vi "Get Common Property Values.vi"(8 "Error In":errorcluster, 11 "Data Channel  Ref in":T2 format="%.0x") -> (0 "error out":errorcluster, 2 "Array Out":T1[](array[typedef]), 3 "Data Channel Ref Out":u64)   [LabVIEW 2019, in "Instrument Addon Scripting API Channels Unit Tests.lvclass"]
uses:
  Instrument Addon Scripting API Channels Unit Tests.lvclass
  <vilib>/NI VeriStand/Custom Device API/Custom Device Item Ref.ctl
  APIs/Scripting API/TypeDefs/Array Element.ctl
  Addon/Addon Shared/SubVIs/Constants.vi
  <vilib>/NI/NI VeriStand Advanced SysDef API/_SubVIs/SysDef.Search.GUIDs.vi
  APIs/Scripting API/Instrument Addon Scripting API.lvlib
  <vilib>/NI VeriStand/Custom Device API/Custom Device API.lvlib
  <vilib>/NI/NI VeriStand Advanced SysDef API/SysDef API/Advanced System Definition.lvlib
  Addon/Addon Shared/Instrument Addon Shared.lvlib
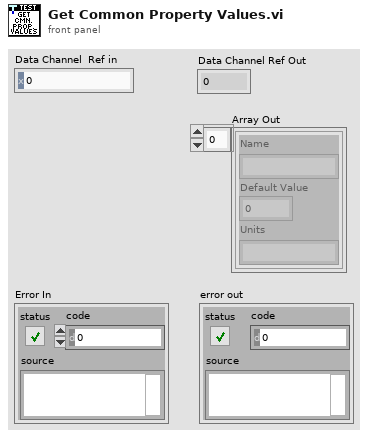
[diagram p1: front panel]
types:
  T1 = typedef "Instrument Addon Scripting API.lvlib/Array Element.ctl" = cluster{"Name":string, "Default Value":dbl, "Units":string}
  T2 = typedef "Custom Device API.lvlib/Custom Device Item Ref.ctl" = u64
  T3 = typedef "Custom Device API.lvlib/Custom Device Channel.ctl" = cluster{"Type":T4, "Units":string, "Default Value":dbl, "Faultable":bool, "Scalable":bool}
  T4 = typedef "Custom Device API.lvlib/Custom Device Channel Type.ctl" = enum16{"Input", "Output"}
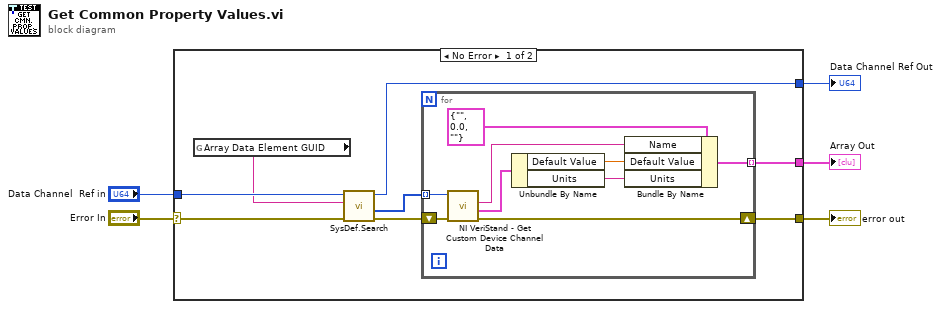
[diagram p0: block diagram]
diagram:
  n1 = case shown="No Error" "Error In" {
    selector: "Error In" -> [w7 w24]
    tunnel: "Data Channel  Ref in" -> [w13 w23]
    tunnel: [w12 _] -> w4
    tunnel: [w11 w23] -> w3
    tunnel: [w10 w24] -> w2
    frame No Error {
      n2 = global read "Constants.vi" "Array Data Element GUID"() -> (w6:string)
      n3 = call-poly <vilib>:"SysDef.Search.vi"("error in (no error)"=w7, "GUID"=w6, "nodeID"=w13) -> ("error out"=w8:errorcluster, "Values Out"=w9:u64[], "nodeID out"=w11:u64)  [unwired: 5 in, 1 out]
      n4 = for {
        shift-right: [w14] -> w10
        shift-left: w8 -> [w21]
        tunnel: w9 -> [w22] mode=indexing
        tunnel: [w15] -> w12 mode=indexing
        n5 = call <vilib>:"NI VeriStand - Get Custom Device Channel Data.vi"("error in (no error)"=w21, "Channel Ref in"=w22) -> ("error out"=w14:errorcluster, "Channel"=w18:T3, "Channel Name"=w19:string)  [unwired: 4 in, 3 out]
        n6 = Unbundle By Name(w18) -> ("Default Value"=w16:dbl, "Units"=w17:string)
        n7 = Bundle By Name(cluster=T1 {"Name"="", "Default Value"=0.0, "Units"=""} ("Array Element"), "Name"=w19, "Default Value"=w16, "Units"=w17) -> (w15:T1)
      }
    }
    frame Error {
    }
  }
  "Array Out" <- w4
  "Data Channel Ref Out" <- w3
  "error out" <- w2
